vi "test_DeviceManager_Setup.vi"(8 "error in (no error)":errorcluster) -> (0 "error out":errorcluster)   [LabVIEW 2023]
doc: "_____\nCreated using DQMH Event Scripter 7.0.0.1280."
uses:
  Libraries/DeviceManager/DeviceManager.lvlib
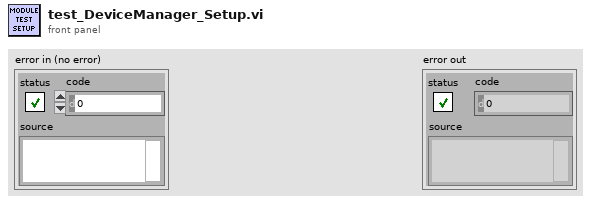
[diagram p1: front panel]
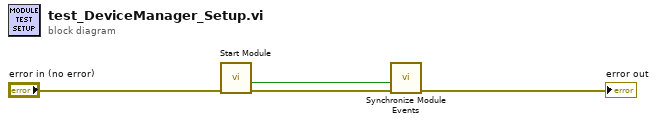
[diagram p0: block diagram]
diagram:
  n1 = call "Start Module.vi"("error in"="error in (no error)") -> ("error out"=w3:errorcluster, "Wait for Event Sync?"=w1:bool)  [unwired: 7 in, 2 out]
  n2 = call "Synchronize Module Events.vi"("error in"=w3, "Wait for Event Sync?"=w1) -> ("error out"=→"error out":errorcluster)  [unwired: 9 in]
